vi "Base Path.vi"() -> (0 "base path out":path)   [LabVIEW 2019]
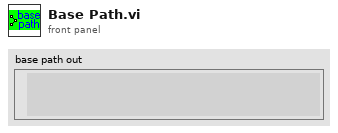
[diagram p1: front panel]
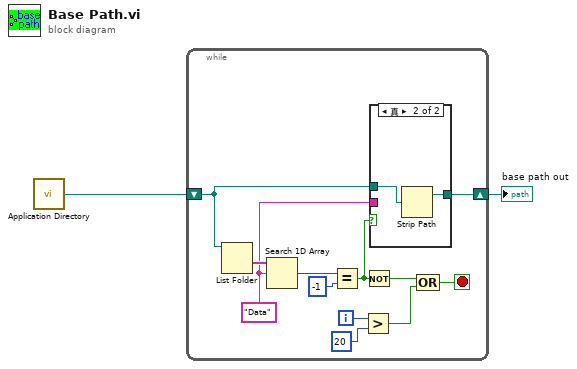
[diagram p0: block diagram]
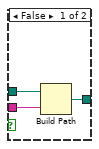
[diagram p2: hidden frame]
diagram:
  n1 = call <vilib>:"Application Directory.vi"() -> ("Application Directory"=w2:path)
  n2 = while "While循环" {
    shift-right: [w10] -> w1
    shift-left: w2 -> [w11]
    i -> [w6]
    stop <- w4 stop-if-true
    w7 = "Data" ("名称或相对路径")
    n3 = List Folder(path=w11) -> (folder names=w14:string[])  [unwired: 3 in, 3 out]
    n4 = Search 1D Array(1D array=w14, element=w7) -> (index of element=w13:i32)  [unwired: 1 in]
    n5 = Equal?(x=w13, y=-1) -> (x = y?=w9:bool)
    n6 = Greater?(x=w6, y=20) -> (0:w3:bool)
    n7 = Not(x=w9) -> (.not. x?=w8:bool)
    n8 = case "条件结构" shown="真" w9 {
      tunnel: w11 -> [w17 w19]
      tunnel: [w15 w18] -> w10
      tunnel: w7 -> [w16 _]
      frame False {
        n9 = Build Path(base path=w17, name or relative path=w16) -> (appended path=w15:path)
      }
      frame True {
        n10 = Strip Path(path=w19) -> (stripped path=w18:path)  [unwired: 1 out]
      }
    }
    n11 = Compound Arithmetic op=OR ("复合运算")(w8, w3) -> (w4:bool)
  }
  "base path out" <- w1
